vi "Excel_Save_Workbook.vi"(0 "Excel._Workbook":refnum<k7>, 5 "password":string, 7 "path":string, 11 "error in (no error)":errorcluster) -> (15 "error out":errorcluster)   [LabVIEW 2020, in "NI_ReportGenerationToolkit.lvlib"]
uses:
  <vilib>/addons/_office/NI_ReportGenerationToolkit.lvlib
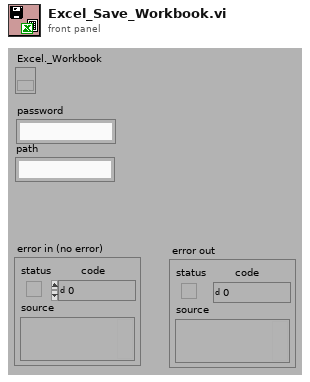
[diagram p1: front panel]
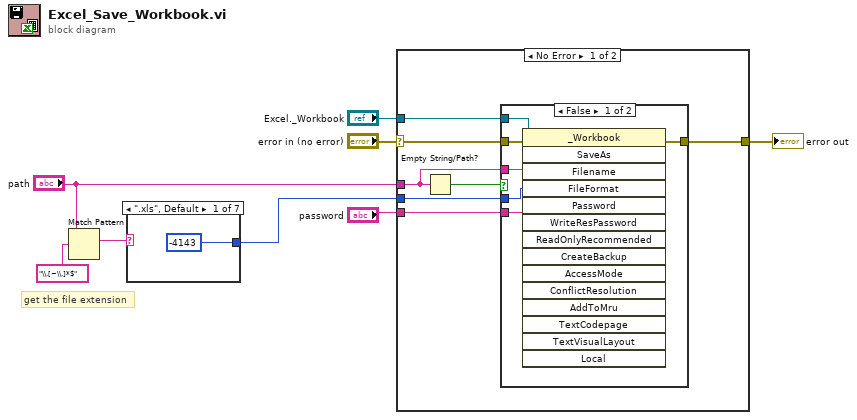
[diagram p0: block diagram]
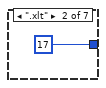
[diagram p2: hidden frame]
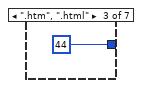
[diagram p3: hidden frame]
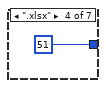
[diagram p4: hidden frame]
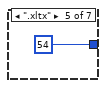
[diagram p5: hidden frame]
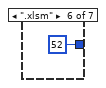
[diagram p6: hidden frame]
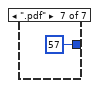
[diagram p7: hidden frame]
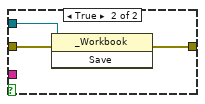
[diagram p8: hidden frame]
diagram:
  # "get the file extension"
  n1 = Match Pattern(string="path", regular expression="\\.[~\\.]*$") -> (match substring=w4:string)  [unwired: 4 out]
  n2 = case shown="\".xls\", Default" w4 {
    tunnel: [-4143 17 44 51 54 52 57] -> w1
    frame ".xls", Default {
    }
    frame ".xlt" {
    }
    frame ".htm", ".html" {
    }
    frame ".xlsx" {
    }
    frame ".xltx" {
    }
    frame ".xlsm" {
    }
    frame ".pdf" {
    }
  }
  n3 = case shown="No Error" "error in (no error)" {
    selector: "error in (no error)" -> [w17 w32]
    tunnel: [w22 w32] -> w8
    tunnel: "Excel._Workbook" -> [w21 _]
    tunnel: "path" -> [w20 _]
    tunnel: "password" -> [w18 _]
    tunnel: w1 -> [w16 _]
    frame No Error {
      n4 = Empty String/Path?(string/path=w20) -> (empty?=w19:bool)
      n5 = case shown="False" w19 {
        tunnel: w21 -> [w26 w31]
        tunnel: w17 -> [w28 w30]
        tunnel: [w27 w29] -> w22
        tunnel: w20 -> [w25 _]
        tunnel: w18 -> [w24 _]
        tunnel: w16 -> [w23 _]
        frame False {
          n6 = invoke class="_Workbook" method="SaveAs"(reference=w26, error in=w28, "Filename"=w25, "FileFormat"=w23, "WriteResPassword"=w24) -> (error out=w27:errorcluster)  [unwired: 10 in, 14 out]
        }
        frame True {
          n7 = invoke class="_Workbook" method="Save"(reference=w31, error in=w30) -> (error out=w29:errorcluster)  [unwired: 1 in, 2 out]
        }
      }
    }
    frame Error {
    }
  }
  "error out" <- w8
